vi "AppendSheet.vi"(8 "error in (no error)":errorcluster, 10 "Name":string, 11 "Excel Interface in":refnum<class "Excel Interface.lvclass">) -> (0 "error out":errorcluster, 2 "Excel Sheet out":refnum<class "Excel Sheet.lvclass">, 3 "Excel Interface out":refnum<class "Excel Interface.lvclass">)   [LabVIEW 2016, in "Excel Interface.lvclass"]
uses:
  Excel Interface.lvclass
  Excel Sheet/Excel Sheet.lvclass
  Excel Interface.lvclass/Excel Interface.ctl
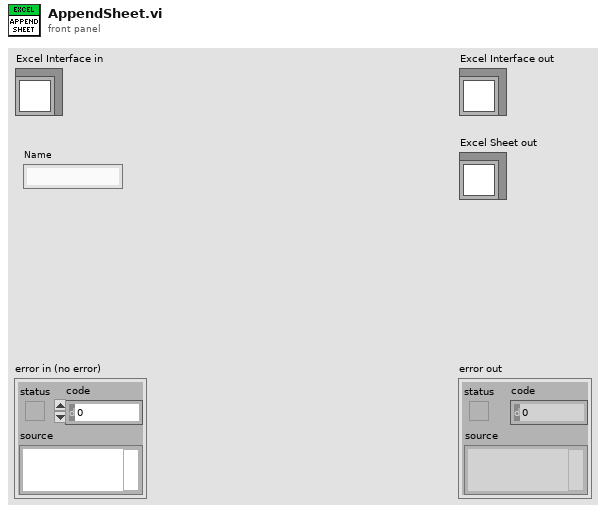
[diagram p1: front panel]
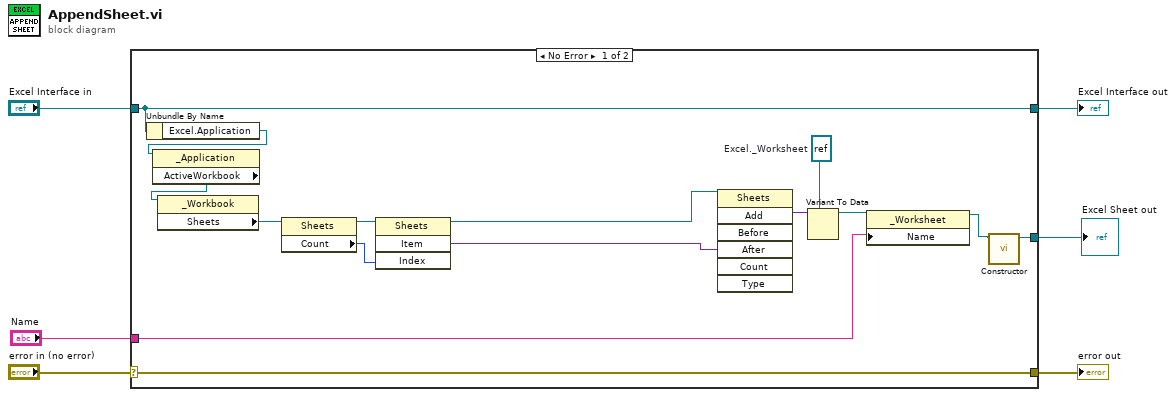
[diagram p0: block diagram]
diagram:
  n1 = case shown="No Error" "error in (no error)" {
    selector: "error in (no error)" -> [w21 w23]
    tunnel: [w21 w23] -> w5
    tunnel: [w18 w22] -> w3
    tunnel: "Excel Interface in" -> [w18 w22]
    tunnel: [w16 _] -> w2
    tunnel: "Name" -> [w13 _]
    frame No Error {
      w17 = refnum<k7> refnum  # Excel._Worksheet
      n2 = Unbundle By Name(w18) -> ("Excel.Application"=w19:refnum<k7>)
      n3 = property class="_Application"(reference=w19) -> ("ActiveWorkbook"=w20:refnum<k7>)  [unwired: 1 in, 2 out]
      n4 = property class="_Workbook"(reference=w20) -> ("Sheets"=w11:refnum<k7>)  [unwired: 1 in, 2 out]
      n5 = property class="Sheets"(reference=w11) -> (reference out=w10:refnum<k7>, "Count"=w9:i32)  [unwired: 1 in, 1 out]
      n6 = invoke class="Sheets" method="Item"(reference=w10, "Index"=w9) -> (reference out=w7:refnum<k7>, "Item"=w8:variant)  [unwired: 2 in, 2 out]
      n7 = invoke class="Sheets" method="Add"(reference=w7, "After"=w8) -> ("Add"=w12:variant)  [unwired: 5 in, 6 out]
      n8 = Variant To Data(type=w17, Variant=w12) -> (data=w15:refnum<k7>)  [unwired: 1 in, 1 out]
      n9 = property class="_Worksheet"(reference=w15, "Name"=w13) -> (reference out=w14:refnum<k7>)  [unwired: 1 in, 1 out]
      n10 = call "Constructor.vi"("Worksheet"=w14) -> ("Excel Sheet out"=w16:refnum<class "Excel Sheet.lvclass">)  [unwired: 10 in]
    }
    frame Error {
    }
  }
  "error out" <- w5
  "Excel Interface out" <- w3
  "Excel Sheet out" <- w2
